vi "Append Popup.vi"(8 "error in (no error)":errorcluster caption="错误输入（无错误）", 10 "PopupRef":refnum<vi>, 11 "Popup 输入":refnum<class "Popup.lvclass"> caption="DNL_LabVIEW Object in") -> (0 "error out":errorcluster caption="错误输出", 3 "Popup 输出":refnum<class "Popup.lvclass"> caption="DNL_LabVIEW Object out")   [LabVIEW 2017, in "Popup.lvclass"]
uses:
  Popup.lvclass
  Popup.lvclass/Popup.ctl
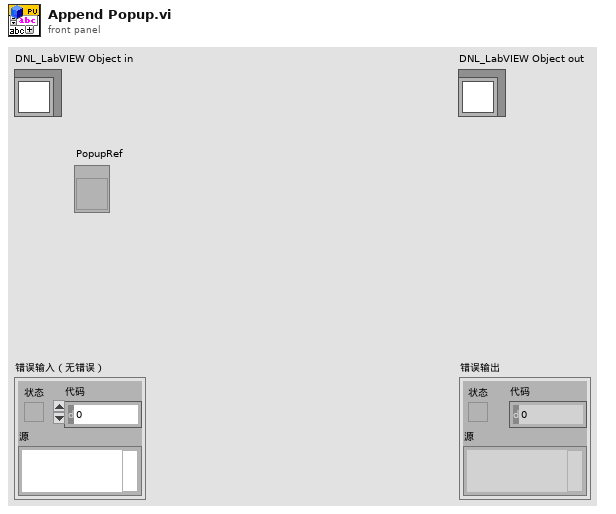
[diagram p1: front panel]
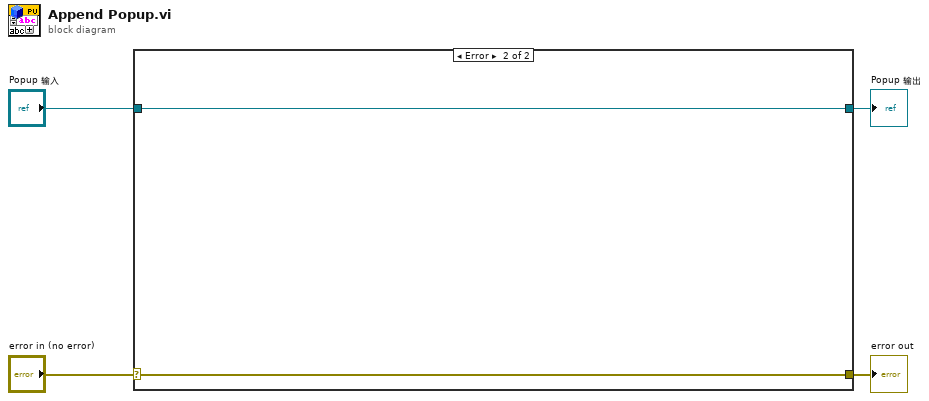
[diagram p0: block diagram]
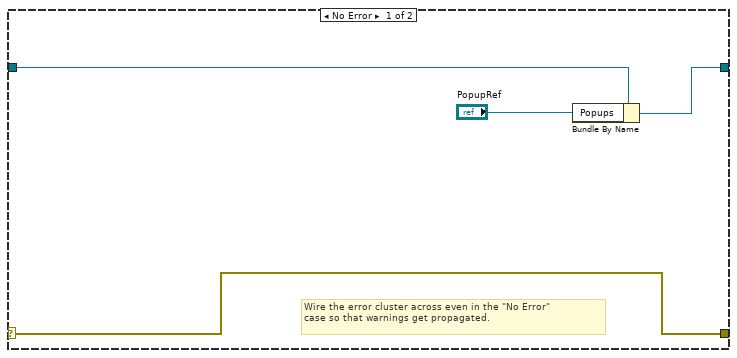
[diagram p2: hidden frame]
diagram:
  n1 = case shown="Error" "error in (no error)" {
    selector: "error in (no error)" -> [w5 w10]
    tunnel: [w5 w10] -> w3
    tunnel: [w8 w9] -> w1
    tunnel: "Popup 输入" -> [w7 w9]
    frame No Error {
      # "Wire the error cluster across even in the \"No Error\"\ncase so that warnings get propagated."
      n2 = Bundle By Name(cluster=w7, "Popups"="PopupRef") -> (w8:refnum<class "Popup.lvclass">)
    }
    frame Error {
    }
  }
  "error out" <- w3
  "Popup 输出" <- w1
